vi "automaticPowerSupplySignal_final_final.vi"() -> ()   [LabVIEW 2022 SP3]
uses:
  <vilib>/DAQmx/read.llb/DAQmx Read (Analog 1D DBL NChan 1Samp).vi
  <vilib>/DAQmx/write.llb/DAQmx Write (Digital Bool 1Line 1Point).vi
  <vilib>/DAQmx/create/channels.llb/DAQmx Create Channel (DO-Digital Output).vi
  <vilib>/DAQmx/create/channels.llb/DAQmx Create Channel (AI-Voltage-Basic).vi
  <vilib>/DAQmx/miscellaneous.llb/DAQmx Fill In Error Info.vi
panel:
  in  "Physical Channels":tag
  in  "lines":tag
  in  "Power Supply":refnum<visa-resource-name>
  out "Gauge 2":dbl(knob) scale=-90.0..90.0
  out "Gauge":dbl(knob) scale=90.0..-90.0
  out "FULL FOLDED":bool
  out "TEMPERATURE SENSOR VOLTAGE":dbl format="%#_3g"
  out "Numeric":dbl
  out "Waveform Chart 3":dbl(graph)
  out "GYRASCOPE ANGLE":dbl format="%#_3g"
  out "RING FINGER ANGLE":dbl format="%#_3g"
  out "MIDLLE FINGER ANGLE":dbl format="%#_3g"
  out "STATUS":bool
  out "SPEED 3":bool
  out "SPEED 2":bool
  out "SPEED 1":bool
  out "FULL FOLDED":bool
  out "REST":bool
  out "REST":bool
  out "FACING RIGHT":bool
  out "REST":bool
  out "FACING LEFT":bool
  out "Gyroscope Position":dbl
  out "Finger 2 Position":dbl
  out "Finger 1 Position":dbl
  in  "stop":bool
  # "PALM POSITION:"
  # "MEASURED POSITIONS OF BEND ANGLE FOR FINGERS"
  # "WINDOW"
  # "MIDDLE FINGER"
  # "RING FINGER"
  # "CEILING FAN REALTIME SPEED"
  # "These two guages display the realtime angle of the fingers. The angle the sensor glove is caliberated for both fingers seperately. The angle has a range of about 90 degrees."
  # "SPEED 2"
  # "MIDDLE FINGER POSITION:"
  # "This Idicates the running conditions of the ceiling fan. The user can either increase or decrease the speed."
  # "RING FINGER POSITION:"
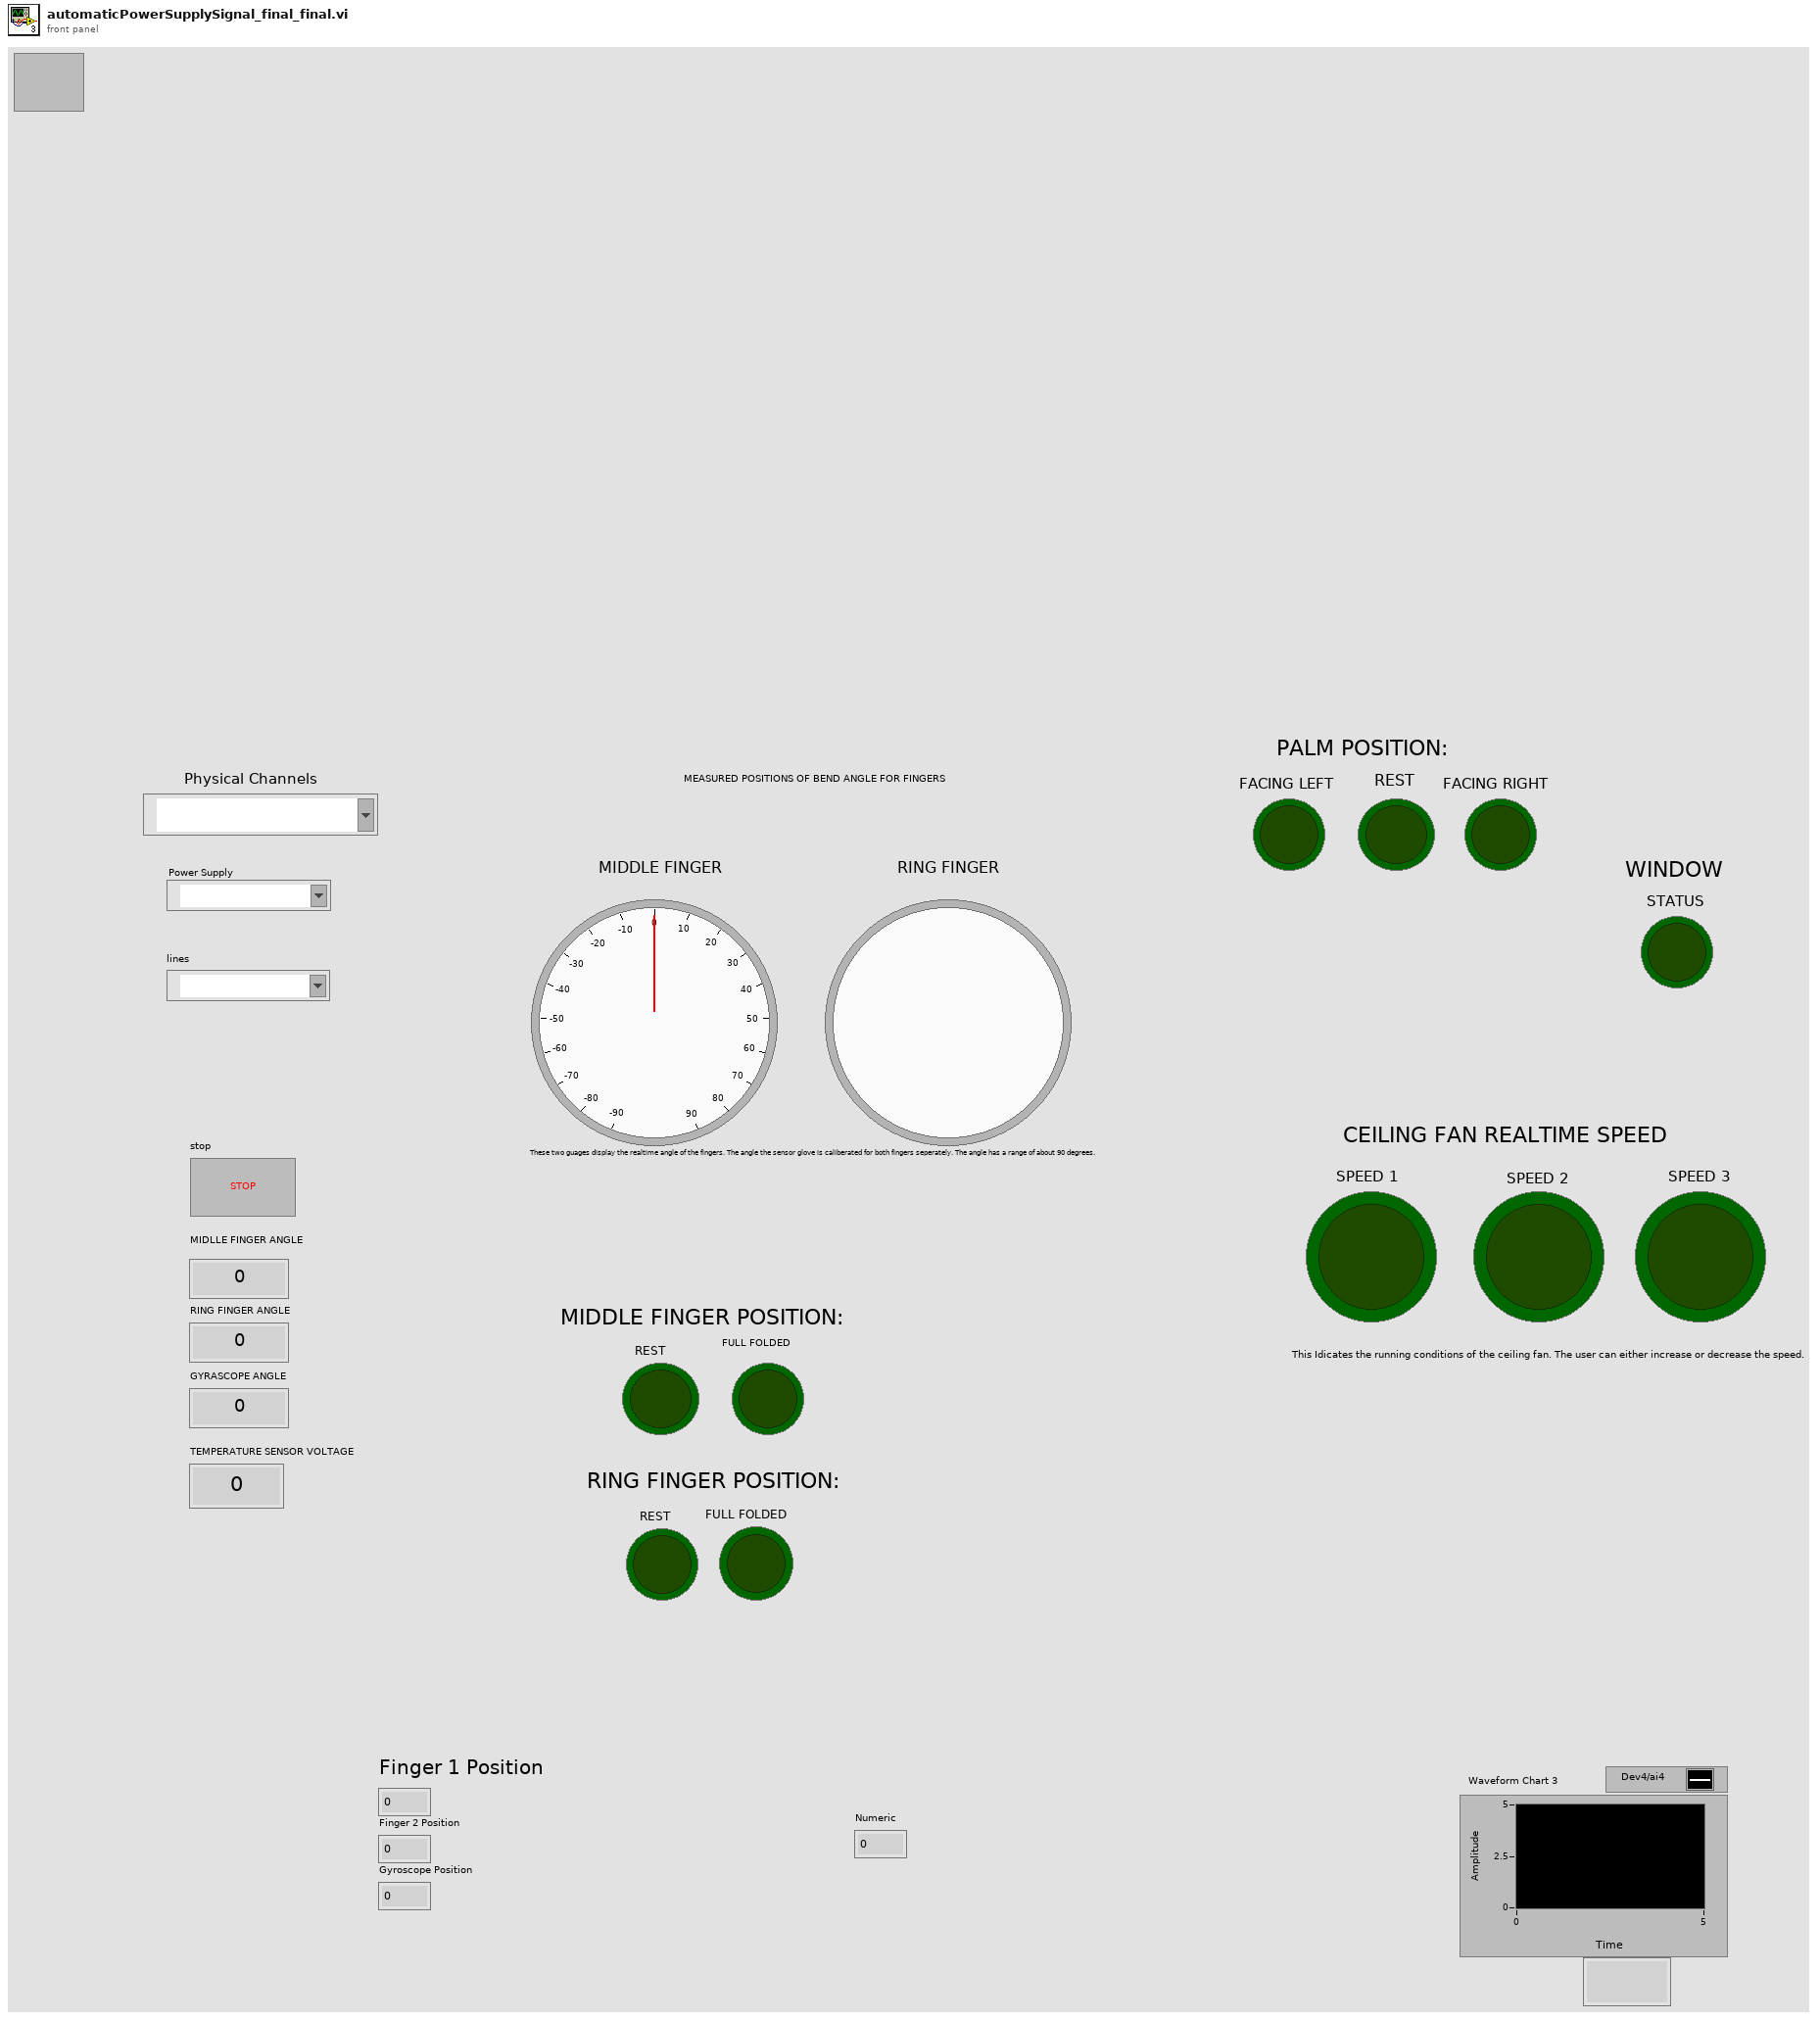
[diagram p1: front panel]
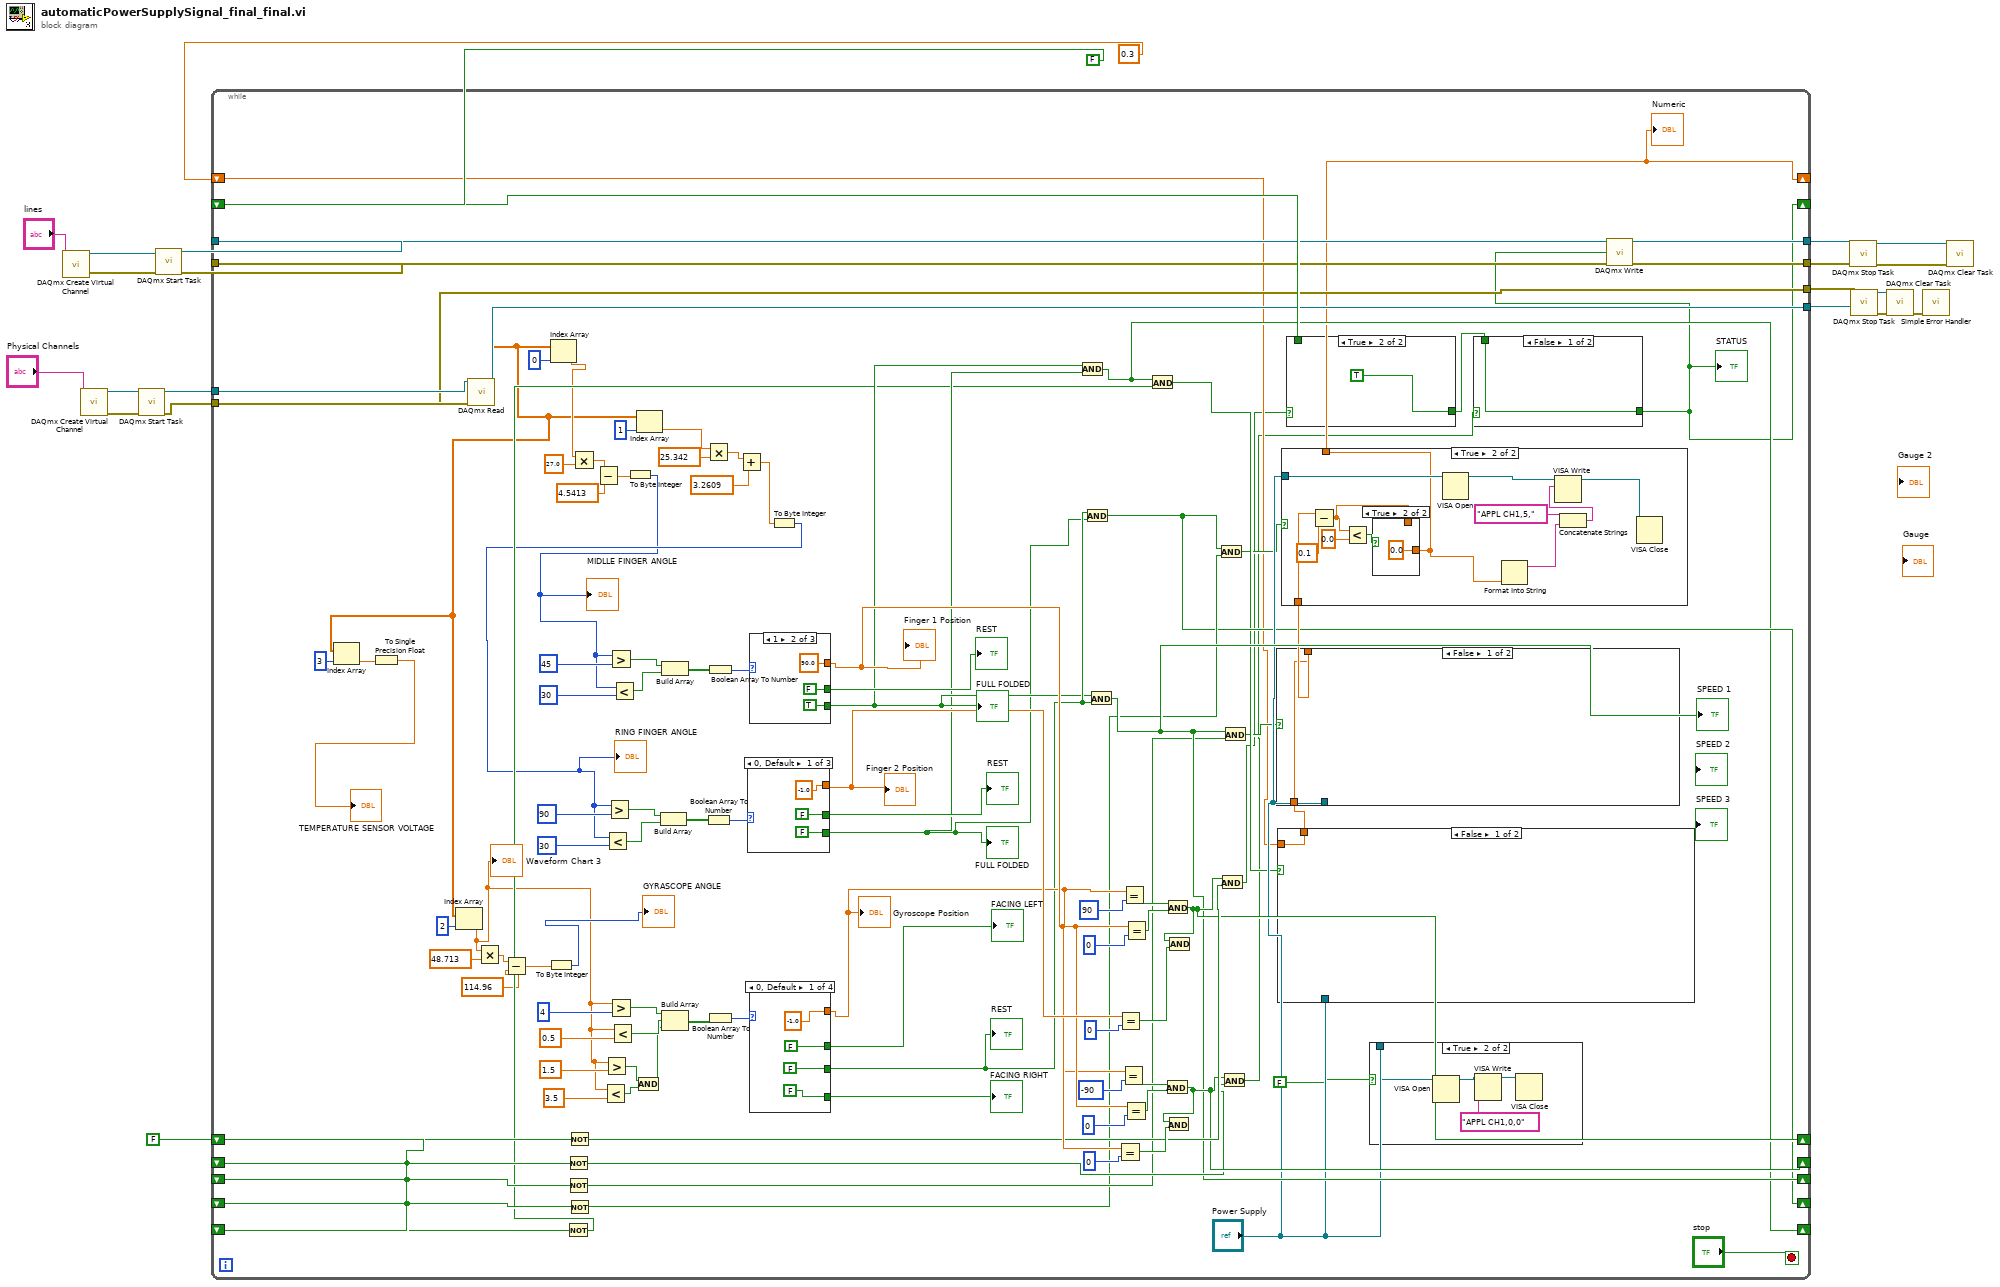
[diagram p0: block diagram]
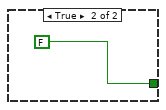
[diagram p2: hidden frame]
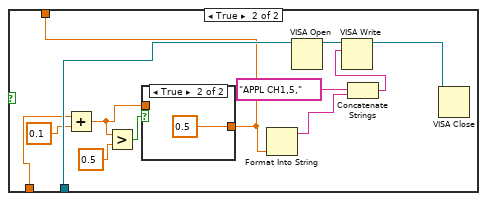
[diagram p6: hidden frame]
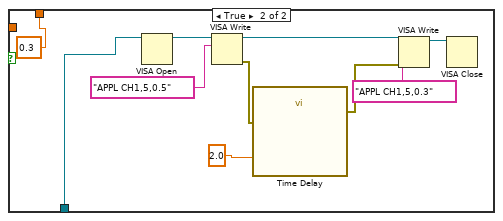
[diagram p9: hidden frame]
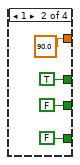
[diagram p10: hidden frame]
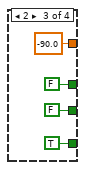
[diagram p11: hidden frame]
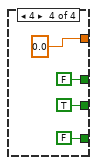
[diagram p12: hidden frame]
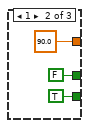
[diagram p13: hidden frame]
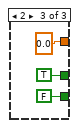
[diagram p14: hidden frame]
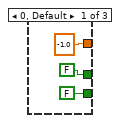
[diagram p15: hidden frame]
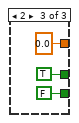
[diagram p16: hidden frame]
diagram:
  w21 = FALSE
  n1 = call-poly <vilib>:"DAQmx Create Virtual Channel.vi"("lines"="lines") -> ("task out"=w19:refnum<k21>, "error out"=w12:errorcluster)  [unwired: 13 in]
  n2 = call-poly <vilib>:"DAQmx Create Virtual Channel.vi"("physical channels"="Physical Channels") -> ("task out"=w10:refnum<k21>, "error out"=w9:errorcluster)  [unwired: 13 in]
  n3 = call <vilib>:"DAQmx Start Task.vi"("task/channels in"=w10, "error in"=w9) -> ("task out"=w7:refnum<k21>, "error out"=w2:errorcluster)  [unwired: 12 in]
  n4 = call <vilib>:"DAQmx Start Task.vi"("task/channels in"=w19, "error in"=w12) -> ("task out"=w18:refnum<k21>, "error out"=w13:errorcluster)  [unwired: 12 in]
  n5 = while {
    shift-right: [w83] -> _
    shift-left: w21 -> [w88]
    shift-right: [w85] -> _
    shift-left: w21 -> [w86]
    shift-right: [w80] -> _
    shift-left: w21 -> [w82]
    shift-right: [w33] -> _
    shift-left: 0.3 -> [w31]
    shift-right: [w68] -> _
    shift-left: w21 -> [w78]
    shift-right: [w67] -> _
    shift-left: w21 -> [w72]
    shift-right: [w28] -> _
    shift-left: FALSE -> [w69]
    tunnel: w18 -> [w66]
    tunnel: [w65] -> w17
    tunnel: [w64] -> w14
    tunnel: w13 -> [w63]
    tunnel: w7 -> [w62]
    tunnel: [w61] -> w3
    tunnel: w2 -> [w60]
    tunnel: [w59] -> w1
    stop <- "stop" stop-if-true
    n6 = call-poly <vilib>:"DAQmx Read.vi"("task/channels in"=w62, "error in"=w60) -> ("task out"=w61:refnum<k21>, "data"=w26:dbl[], "error out"=w59:errorcluster)  [unwired: 11 in]
    n7 = Index Array(array=w26, index=3) -> (element=w24:dbl)
    n8 = To Single Precision Float(number=w24) -> (single precision float=→"TEMPERATURE SENSOR VOLTAGE":sgl)
    n9 = Index Array(array=w26, index=2) -> (element=w37:dbl)
    "Waveform Chart 3" <- w37
    n10 = Multiply(x=w37, y=48.713) -> (x*y=w41:dbl)
    n11 = Subtract(x=w41, y=114.96) -> (x-y=w38:dbl)
    n12 = To Byte Integer(number=w38) -> (8bit integer=→"GYRASCOPE ANGLE":i8)
    n13 = Index Array(array=w26, index=0 ("index (row)")) -> (element=w55:dbl)
    n14 = Not(x=w72) -> (.not. x?=w71:bool)
    n15 = Not(x=w86) -> (.not. x?=w81:bool)
    n16 = Not(x=w82) -> (.not. x?=w77:bool)
    n17 = Not(x=w88) -> (.not. x?=w87:bool)
    n18 = Not(x=w78) -> (.not. x?=w73:bool)
    n19 = Multiply(x=w55, y=27.0) -> (x*y=w53:dbl)
    n20 = Subtract(x=w53, y=4.5413) -> (x-y=w45:dbl)
    n21 = Less?(x=w37, y=3.5) -> (x < y?=w111:bool)
    n22 = Greater?(x=w37, y=1.5) -> (0:w112:bool)
    n23 = Greater?(x=w37, y=4) -> (0:w122:bool)
    n24 = Less?(x=w37, y=0.5) -> (x < y?=w119:bool)
    n25 = To Byte Integer(number=w45) -> (8bit integer=w44:i8)
    "MIDLLE FINGER ANGLE" <- w44
    n26 = Greater?(x=w44, y=45) -> (0:w129:bool)
    n27 = Less?(x=w44, y=30) -> (x < y?=w117:bool)
    n28 = And(x=w112, y=w111) -> (x .and. y?=w110:bool)
    n29 = Index Array(array=w26, index=1 ("index (row)")) -> (element=w50:dbl)
    n30 = Build Array(w129, w117) -> (w128:bool[])
    n31 = Build Array(w122, w119, w110) -> (w121:bool[])
    n32 = Multiply(x=w50, y=25.342) -> (x*y=w48:dbl)
    n33 = Boolean Array To Number(Boolean array=w128) -> (number=w97:u32)
    n34 = Boolean Array To Number(Boolean array=w121) -> (number=w109:u32)
    n35 = Add(x=w48, y=3.2609) -> (x+y=w47:dbl)
    n36 = case shown="1" w97 {
      tunnel: [-1.0 ("Finger 1 Position") 90.0 ("Finger 1 Position") 0.0 ("Finger 1 Position")] -> w89
      tunnel: [FALSE ("F-REST") FALSE ("F-REST") TRUE ("F-REST")] -> w106
      tunnel: [FALSE ("F-FULL FOLDED") TRUE ("F-FULL FOLDED") FALSE ("F-FULL FOLDED")] -> w75
      frame 0, Default {
      }
      frame 1 {
      }
      frame 2 {
      }
    }
    "Finger 1 Position" <- w89
    "REST" <- w106
    "FULL FOLDED" <- w75
    n37 = case shown="0, Default" w109 {
      tunnel: [-1.0 ("Finger 1 Position") 90.0 ("Finger 1 Position") -90.0 ("Finger 1 Position") 0.0 ("Finger 1 Position")] -> w84
      tunnel: [FALSE ("FACING LEFT") TRUE ("FACING LEFT") FALSE ("FACING LEFT") FALSE ("FACING LEFT")] -> w108
      tunnel: [FALSE ("REST") FALSE ("REST") FALSE ("REST") TRUE ("REST")] -> w79
      tunnel: [FALSE ("FACING RIGHT") FALSE ("FACING RIGHT") TRUE ("FACING RIGHT") FALSE ("FACING RIGHT")] -> w107
      frame 0, Default {
      }
      frame 1 {
      }
      frame 2 {
      }
      frame 4 {
      }
    }
    "Gyroscope Position" <- w84
    "FACING LEFT" <- w108
    "REST" <- w79
    "FACING RIGHT" <- w107
    n38 = To Byte Integer(number=w47) -> (8bit integer=w46:i8)
    "RING FINGER ANGLE" <- w46
    n39 = Less?(x=w46, y=30) -> (x < y?=w115:bool)
    n40 = Greater?(x=w46, y=90) -> (0:w125:bool)
    n41 = Build Array(w125, w115) -> (w126:bool[])
    n42 = Boolean Array To Number(Boolean array=w126) -> (number=w127:u32)
    n43 = case shown="0, Default" w127 {
      tunnel: [-1.0 ("Finger 1 Position") 90.0 ("Finger 1 Position") 0.0 ("Finger 1 Position")] -> w101
      tunnel: [FALSE ("M-REST") FALSE ("M-REST") TRUE ("M-REST")] -> w105
      tunnel: [FALSE ("M-FULL FOLDED") TRUE ("M-FULL FOLDED") FALSE ("M-FULL FOLDED")] -> w74
      frame 0, Default {
      }
      frame 1 {
      }
      frame 2 {
      }
    }
    "Finger 2 Position" <- w101
    "REST" <- w105
    "FULL FOLDED" <- w74
    n44 = And(x=w75, y=w74) -> (x .and. y?=w67:bool)
    n45 = And(x=w79, y=w74) -> (x .and. y?=w68:bool)
    n46 = And(x=w75, y=w79) -> (x .and. y?=w80:bool)
    "SPEED 1" <- w80
    n47 = Equal?(x=w89, y=0) -> (x = y?=w90:bool)
    n48 = Equal?(x=w101, y=0) -> (x = y?=w98:bool)
    n49 = Equal?(x=w84, y=-90) -> (x = y?=w92:bool)
    n50 = Equal?(x=w84, y=90) -> (x = y?=w100:bool)
    n51 = Equal?(x=w89, y=0) -> (x = y?=w91:bool)
    n52 = Equal?(x=w89, y=0) -> (x = y?=w99:bool)
    n53 = And(x=w67, y=w71) -> (x .and. y?=w36:bool)
    n54 = And(x=w92, y=w91) -> (x .and. y?=w85:bool)
    n55 = And(x=w100, y=w99) -> (x .and. y?=w83:bool)
    n56 = And(x=w85, y=w90) -> ()  [unwired: 1 out]
    n57 = And(x=w83, y=w98) -> ()  [unwired: 1 out]
    n58 = And(x=w68, y=w73) -> (x .and. y?=w35:bool)
    n59 = And(x=w83, y=w87) -> (x .and. y?=w30:bool)
    n60 = And(x=w85, y=w81) -> (x .and. y?=w27:bool)
    n61 = And(x=w80, y=w77) -> (x .and. y?=w34:bool)
    n62 = case shown="False" w36 {
      tunnel: "Power Supply" -> [_ w175]
      tunnel: [w169 0.3 ("x")] -> w32
      tunnel: w31 -> [w169 _]
      frame False {
      }
      frame True {
        n63 = VISA Open(VISA resource name=w175) -> (VISA resource name=w179:refnum<visa-resource-name>)  [unwired: 4 in, 1 out]
        n64 = VISA Write(VISA resource name=w179, write buffer="APPL CH1,5,0.5") -> (VISA resource name out=w174:refnum<visa-resource-name>, error out=w173:errorcluster)  [unwired: 1 in, 1 out]
        n65 = call "Time Delay"("error in (no error)"=w173, "Delay Time (s)"=2.0) -> ("error out"=w171:errorcluster)  [unwired: 9 in]
        n66 = VISA Write(VISA resource name=w174, write buffer="APPL CH1,5,0.3", error in (no error)=w171) -> (VISA resource name out=w178:refnum<visa-resource-name>)  [unwired: 2 out]
        n67 = VISA Close(VISA resource name=w178) -> ()  [unwired: 1 in, 1 out]
      }
    }
    n68 = case shown="False" w34 {
      tunnel: "Power Supply" -> [_ w161]
      tunnel: [w150 w153] -> w76
      tunnel: w32 -> [w150 w151]
      frame False {
      }
      frame True {
        n69 = Add(x=w151, y=0.1) -> (x+y=w152:dbl)
        n70 = Greater?(x=w152, y=0.5) -> (0:w154:bool)
        n71 = case shown="True" w154 {
          tunnel: [w163 0.5] -> w153
          tunnel: w152 -> [w163 _]
          frame False {
          }
          frame True {
          }
        }
        n72 = Format Into String(w153) -> (resulting string=w156:string)  [unwired: 3 in, 1 out]
        n73 = VISA Open(VISA resource name=w161) -> (VISA resource name=w162:refnum<visa-resource-name>)  [unwired: 4 in, 1 out]
        n74 = Concatenate Strings("APPL CH1,5," ("write buffer"), w156) -> (w158:string)
        n75 = VISA Write(VISA resource name=w162, write buffer=w158) -> (VISA resource name out=w160:refnum<visa-resource-name>)  [unwired: 1 in, 2 out]
        n76 = VISA Close(VISA resource name=w160) -> ()  [unwired: 1 in, 1 out]
      }
    }
    n77 = case shown="True" w35 {
      tunnel: "Power Supply" -> [_ w143]
      tunnel: w76 -> [w135 w142]
      tunnel: [w135 w137] -> w33
      frame False {
      }
      frame True {
        n78 = Subtract(x=w142, y=0.1) -> (x-y=w136:dbl)
        n79 = Less?(x=w136, y=0.0) -> (x < y?=w138:bool)
        n80 = case shown="True" w138 {
          tunnel: [w148 0.0] -> w137
          tunnel: w136 -> [w148 _]
          frame False {
          }
          frame True {
          }
        }
        n81 = VISA Open(VISA resource name=w143) -> (VISA resource name=w147:refnum<visa-resource-name>)  [unwired: 4 in, 1 out]
        n82 = Format Into String(w137) -> (resulting string=w140:string)  [unwired: 3 in, 1 out]
        n83 = Concatenate Strings("APPL CH1,5," ("write buffer"), w140) -> (w144:string)
        n84 = VISA Write(VISA resource name=w147, write buffer=w144) -> (VISA resource name out=w146:refnum<visa-resource-name>)  [unwired: 1 in, 2 out]
        n85 = VISA Close(VISA resource name=w146) -> ()  [unwired: 1 in, 1 out]
      }
    }
    "Numeric" <- w33
    n86 = case shown="True" w30 {
      tunnel: w69 -> [w133 _]
      tunnel: [w133 TRUE] -> w29
      frame False {
      }
      frame True {
      }
    }
    n87 = case shown="True" FALSE {
      tunnel: "Power Supply" -> [_ w165]
      frame False {
      }
      frame True {
        n88 = VISA Open(VISA resource name=w165) -> (VISA resource name=w166:refnum<visa-resource-name>)  [unwired: 4 in, 1 out]
        n89 = VISA Write(VISA resource name=w166, write buffer="APPL CH1,0,0") -> (VISA resource name out=w168:refnum<visa-resource-name>)  [unwired: 1 in, 2 out]
        n90 = VISA Close(VISA resource name=w168) -> ()  [unwired: 1 in, 1 out]
      }
    }
    n91 = case shown="False" w27 {
      tunnel: w29 -> [w131 _]
      tunnel: [w131 FALSE] -> w28
      frame False {
      }
      frame True {
      }
    }
    "STATUS" <- w28
    n92 = call-poly <vilib>:"DAQmx Write.vi"("task/channels in"=w66, "data"=w28, "error in"=w63) -> ("task out"=w65:refnum<k21>, "error out"=w64:errorcluster)  [unwired: 10 in, 1 out]
  }
  n93 = call <vilib>:"DAQmx Stop Task.vi"("task/channels in"=w17, "error in"=w14) -> ("task out"=w16:refnum<k21>, "error out"=w15:errorcluster)  [unwired: 12 in]
  n94 = call <vilib>:"DAQmx Stop Task.vi"("task/channels in"=w3, "error in"=w1) -> ("task out"=w6:refnum<k21>, "error out"=w4:errorcluster)  [unwired: 12 in]
  n95 = call <vilib>:"DAQmx Clear Task.vi"("task in"=w6, "error in"=w4) -> ("error out"=w5:errorcluster)  [unwired: 13 in]
  n96 = call <vilib>:"Simple Error Handler.vi"("error in (no error)"=w5) -> ()  [unwired: 4 in, 5 out]
  n97 = call <vilib>:"DAQmx Clear Task.vi"("task in"=w16, "error in"=w15) -> ()  [unwired: 13 in, 1 out]
